vi "VLC - Save Stream.vi"(5 "Media Source":string="rtsp://user:password@*.*.*.*/axis-media/media.amp?videocodec=h264", 7 "Script":string=":sout=#duplicate{dst=display,dst=\"transcode{vcodec=h264,scale=1,soverlay,sfilter={marq{marquee='Enter Text Here %Y-%m-%d %H:%M:%S',position=9}:logo{file='C:\\Users\\artur\\Desktop\\Labview.png',position=5,transparency=255}}}\"}:duplicate{dst=std{access=file,mux=ts,dst='D:\\Video\\LabVIEW_VLC_Script.ts'}}", 11 "error in (no error)":errorcluster) -> (15 "error out":errorcluster)   [LabVIEW 2011]
uses:
  System.Windows.Forms
  <vilib>/Utility/sysdir.llb/System Directory Type.ctl
panel:
  out "Failed":bool
  in  "PictureBox":refnum<k24>(container)
  in  "Snap":bool
  # "http://www.videolan.org/developers/vlc/doc/doxygen/html/modules.html"
  # "Snapshot doesn't work...\nhttps://forum.videolan.org/viewtopic.php?f=14&t=104610"
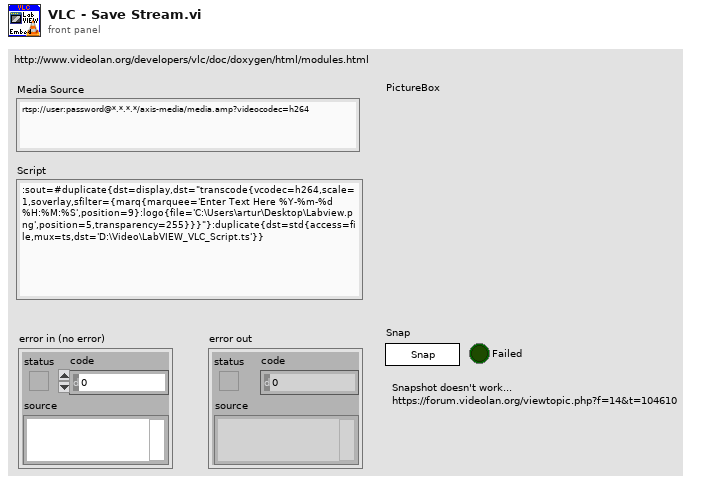
[diagram p1: front panel]
types:
  T1 = typedef "System Directory Type.ctl" = i32
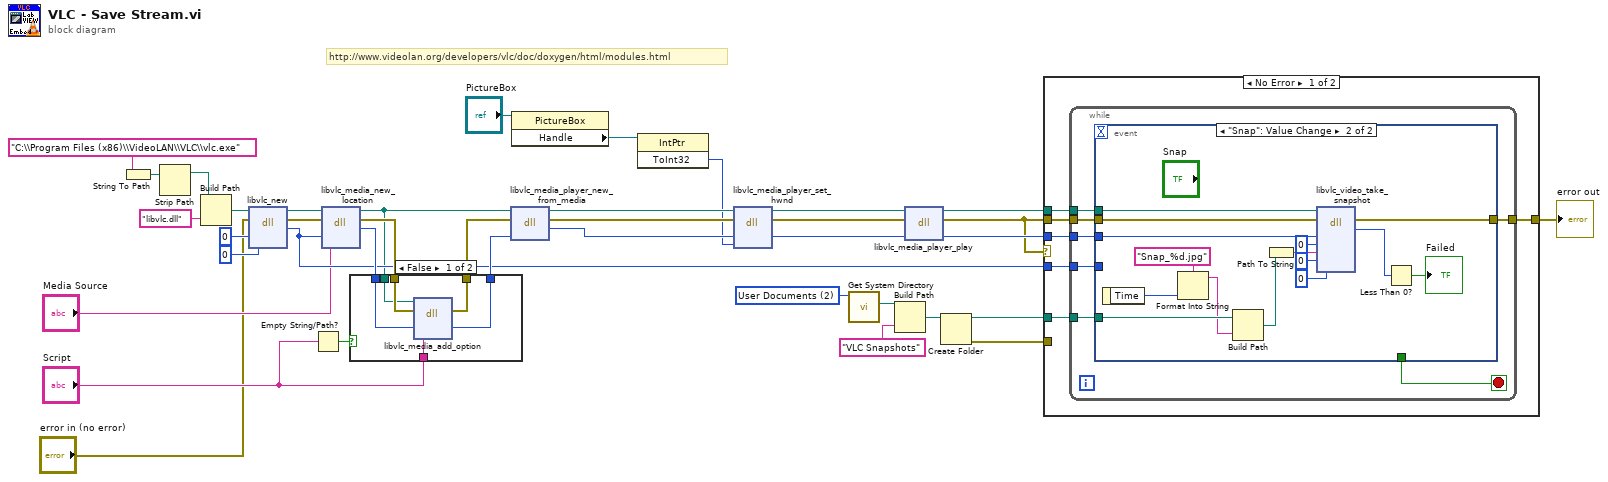
[diagram p0: block diagram]
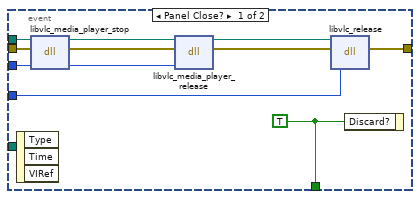
[diagram p2: hidden frame]
diagram:
  w8 = T1 2 items=["User Home"=0, "User Desktop"=1, "User Documents"=2, "User Application Data"=3, "User Preferences"=4, "User Temporary"=5, "Public Documents"=6, "Public Application Data"=7, "Public Preferences"=8, "Public Cache"=13, "System Core Libraries"=9, "System Installed Libraries"=10, "Application Files"=11, "Boot Volume Root"=12] ("system directory type")
  # "http://www.videolan.org/developers/vlc/doc/doxygen/html/modules.html"
  n1 = String To Path(string="C:\\Program Files (x86)\\VideoLAN\\VLC\\vlc.exe") -> (path=w21:path)
  n2 = Strip Path(path=w21) -> (stripped path=w20:path)  [unwired: 1 out]
  n3 = Build Path(base path=w20, name or relative path="libvlc.dll") -> (appended path=w18:path)
  n4 = dll-call lib="C:/Program Files (x86)/VideoLAN/VLC/libvlc.dll" fn="libvlc_new"(path in=w18, error in="error in (no error)", "argc"=i16 0, "argv"=u8 0) -> (path out=w25:path, error out=w28:errorcluster, "return type"=w34:i32)  [unwired: 3 in]
  n5 = Empty String/Path?(string/path="Script") -> (empty?=w15:bool)
  n6 = dll-call lib="C:/Program Files (x86)/VideoLAN/VLC/libvlc.dll" fn="libvlc_media_new_location"(path in=w25, error in=w28, "p_instance"=w34, "path"="Media Source") -> (path out=w12:path, error out=w35:errorcluster, "return type"=w36:i32)  [unwired: 3 in]
  n7 = case shown="False" w15 {
    tunnel: w35 -> [w44 w46]
    tunnel: w36 -> [w43 w45]
    tunnel: [w42 w45] -> w37
    tunnel: [w41 w46] -> w38
    tunnel: "Script" -> [w40 _]
    tunnel: w12 -> [w39 _]
    frame False {
      n8 = dll-call lib="C:/Program Files (x86)/VideoLAN/VLC/libvlc.dll" fn="libvlc_media_add_option"(path in=w39, error in=w44, "p_md"=w43, "ppsz_options"=w40) -> (error out=w41:errorcluster, "p_md"=w42:i32)  [unwired: 3 in, 1 out]
    }
    frame True {
    }
  }
  n9 = dll-call lib="C:/Program Files (x86)/VideoLAN/VLC/libvlc.dll" fn="libvlc_media_player_new_from_media"(path in=w12, error in=w38, "p_md"=w37) -> (path out=w24:path, error out=w31:errorcluster, "return type"=w29:i32)  [unwired: 2 in]
  n10 = property class="PictureBox"(reference="PictureBox") -> ("Handle"=w10:refnum<k24>)  [unwired: 1 in, 2 out]
  n11 = invoke class="IntPtr" method="ToInt32"(reference=w10) -> ("ToInt32"=w9:i32)  [unwired: 2 in, 2 out]
  n12 = dll-call lib="C:/Program Files (x86)/VideoLAN/VLC/libvlc.dll" fn="libvlc_media_player_set_hwnd"(path in=w24, error in=w31, "p_mi"=w29, "drawable"=w9) -> (path out=w23:path, error out=w32:errorcluster, "p_mi"=w30:i32)  [unwired: 3 in]
  n13 = call <vilib>:"Get System Directory.vi"("system directory type"=w8) -> ("system directory"=w7:path)  [unwired: 10 in]
  n14 = Build Path(base path=w7, name or relative path="VLC Snapshots") -> (appended path=w5:path)
  n15 = dll-call lib="C:/Program Files (x86)/VideoLAN/VLC/libvlc.dll" fn="libvlc_media_player_play"(path in=w23, error in=w32, "p_mi"=w30) -> (path out=w22:path, error out=w13:errorcluster, "p_mi"=w33:i32)  [unwired: 2 in]
  n16 = Create Folder(path (use dialog)=w5) -> (created path=w4:path, error out=w3:errorcluster)  [unwired: 2 in, 1 out]
  n17 = case shown="No Error" w13 {
    tunnel: w34 -> [w52 _]
    tunnel: w33 -> [w51 _]
    tunnel: w13 -> [w50 w86]
    tunnel: w22 -> [w49 _]
    tunnel: [w48 w86] -> w14
    tunnel: w4 -> [w47 _]
    tunnel: w3 -> [_ _]
    frame No Error {
      n18 = while {
        tunnel: w52 -> [w59]
        tunnel: w51 -> [w58]
        tunnel: w50 -> [w57]
        tunnel: w49 -> [w56]
        tunnel: [w55] -> w48
        tunnel: w47 -> [w53]
        stop <- w54 stop-if-true
        n19 = event shown="[1] \"Snap\": Value Change" {
          selector: _ -> [_ _]
          dyn-events: _ -> [_ _]
          timeout: _ -> [_ _]
          tunnel: w57 -> [w70 w80]
          tunnel: w58 -> [w69 w78]
          tunnel: w59 -> [w65 _]
          tunnel: w56 -> [w64 w81]
          tunnel: [w61 w79] -> w55
          tunnel: [w60 _] -> w54
          tunnel: w53 -> [_ w75]
          event Panel Close? {
            w60 = TRUE ("Discard?")
            n20 = event-data() -> ()  [unwired: 1 in, 3 out]
            n21 = dll-call lib="C:/Program Files (x86)/VideoLAN/VLC/libvlc.dll" fn="libvlc_media_player_stop"(path in=w64, error in=w70, "p_mi"=w69) -> (path out=w63:path, error out=w68:errorcluster, "p_mi"=w67:i32)  [unwired: 2 in]
            n22 = dll-call lib="C:/Program Files (x86)/VideoLAN/VLC/libvlc.dll" fn="libvlc_media_player_release"(path in=w63, error in=w68, "p_mi"=w67) -> (path out=w62:path, error out=w66:errorcluster)  [unwired: 3 in]
            n23 = dll-call lib="C:/Program Files (x86)/VideoLAN/VLC/libvlc.dll" fn="libvlc_release"(path in=w62, error in=w66, "p_instnace"=w65) -> (error out=w61:errorcluster)  [unwired: 3 in, 1 out]
            n24 = event-data("Discard?"=w60) -> ()  [unwired: 1 in, 1 out]
          }
          event "Snap": Value Change {
            n25 = event-data() -> ("Time"=w77:u32)  [unwired: 1 in]
            n26 = Format Into String(format string="Snap_%d.jpg", w77) -> (resulting string=w74:string)  [unwired: 2 in, 1 out]
            n27 = Build Path(base path=w75, name or relative path=w74) -> (appended path=w73:path)
            n28 = Path To String(path=w73) -> (string=w83:string)
            n29 = dll-call lib="C:/Program Files (x86)/VideoLAN/VLC/libvlc.dll" fn="libvlc_video_take_snapshot"(path in=w81, error in=w80, "p_mi"=w78, "num"=u32 0, "psz_filepath"=w83, "i_width"=u32 0, "i_height"=u32 0) -> (error out=w79:errorcluster, "return type"=w72:i32)  [unwired: 6 in, 1 out]
            n30 = Less Than 0?(x=w72) -> (x < 0?=→"Failed":bool)
          }
        }
      }
    }
    frame Error {
    }
  }
  "error out" <- w14
